vi "DBL.vi"(4 "Value":T1) -> (1 "Constant":refnum<class "Const_I32.lvclass">)   [LabVIEW 2021, in "Const_I32.lvclass"]
uses:
  Const_I32.lvclass
  Type.ctl
  Const_I32.lvclass/Const_I32.ctl
  Properties/Write Value.vi
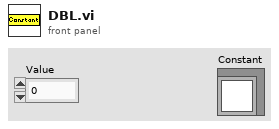
[diagram p1: front panel]
types:
  T1 = typedef "Const_I32.lvclass/Type.ctl" = dbl
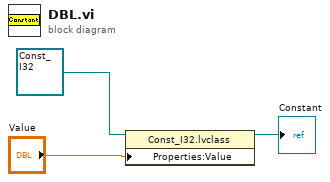
[diagram p0: block diagram]
diagram:
  n1 = property class="Const_I32.lvclass"(reference=refnum<class "Const_I32.lvclass"> refnum ("Constants.lvlib:Numeric.lvclass"), "Properties:Value"="Value") -> (reference out=→"Constant":refnum<class "Const_I32.lvclass">)  [unwired: 1 in, 1 out]
